vi "Create Folder.vi"(8 "error in (no error)":errorcluster caption="Error In", 11 "Path In":path) -> (0 "error out":errorcluster caption="Error Out", 3 "Path Out":path)   [LabVIEW 2020]
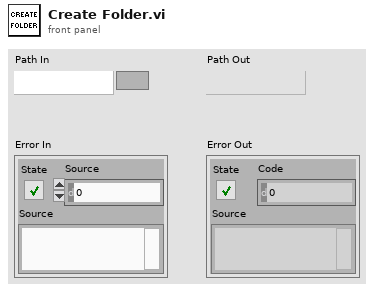
[diagram p1: front panel]
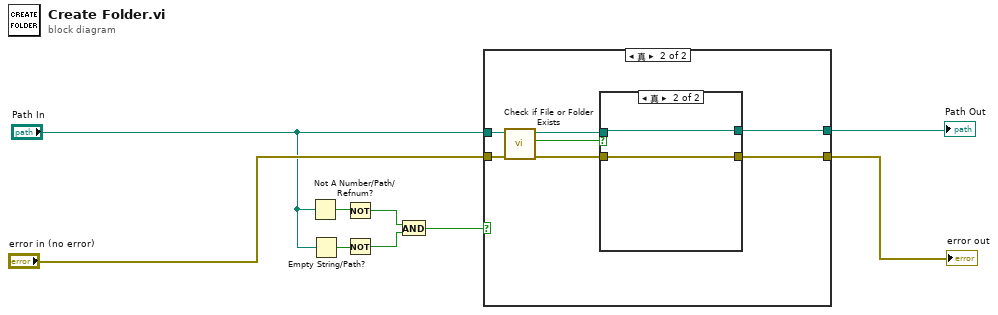
[diagram p0: block diagram]
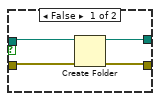
[diagram p3: hidden frame]
diagram:
  n1 = Not A Number/Path/Refnum?(number/path/refnum="Path In") -> (NaN/Path/Refnum?=w6:bool)
  n2 = Empty String/Path?(string/path="Path In") -> (empty?=w5:bool)
  n3 = Not(x=w6) -> (.not. x?=w3:bool)
  n4 = Not(x=w5) -> (.not. x?=w2:bool)
  n5 = And(x=w3, y=w2) -> (x .and. y?=w1:bool)
  n6 = case shown="真" w1 {
    tunnel: [w11 w15] -> w9
    tunnel: "error in (no error)" -> [w10 w14]
    tunnel: [w10 w13] -> w7
    tunnel: "Path In" -> [w11 w12]
    frame False {
    }
    frame True {
      n7 = call <vilib>:"Check if File or Folder Exists.vi"("error in (no error)"=w14, "path"=w12) -> ("error out"=w17:errorcluster, "file or folder exists?"=w16:bool, "dup path"=w18:path)  [unwired: 7 in]
      n8 = case shown="真" w16 {
        tunnel: w18 -> [w21 w24]
        tunnel: w17 -> [w22 w23]
        tunnel: [w20 w24] -> w15
        tunnel: [w19 w23] -> w13
        frame False {
          n9 = Create Folder(path (use dialog)=w21, error in=w22) -> (created path=w20:path, error out=w19:errorcluster)  [unwired: 1 in, 1 out]
        }
        frame True {
        }
      }
    }
  }
  "Path Out" <- w9
  "error out" <- w7
